vi "Init_Robot_State.vi"(8 "error in (no error)":errorcluster) -> (0 "error out":errorcluster, 3 "MotionCtlLoop_Data":T1)   [LabVIEW 2017]
doc: "Initialise robot's position and forward & rotation velocity to 0"
uses:
  Ctl/MotionControlLoop_Data_Cluster.ctl
  Ctl/Current_Position.ctl
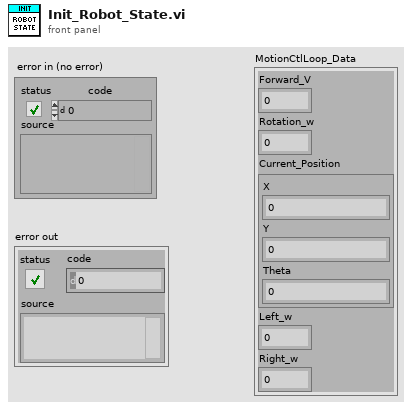
[diagram p1: front panel]
types:
  T1 = typedef "MotionControlLoop_Data_Cluster.ctl" = cluster{"Forward_V":dbl, "Rotation_w":dbl, "Current_Position":T2, "Left_w":dbl, "Right_w":dbl}
  T2 = typedef "Current_Position.ctl" = cluster{"X":dbl, "Y":dbl, "Theta":dbl}
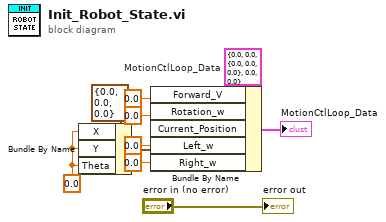
[diagram p0: block diagram]
diagram:
  w10 = 0.0 ("X")
  w2 = T1 {"Forward_V"=0.0, "Rotation_w"=0.0, "Current_Position"={"X"=0.0, "Y"=0.0, "Theta"=0.0}, "Left_w"=0.0, "Right_w"=0.0}  # MotionCtlLoop_Data
  n1 = Bundle By Name(cluster=T2 {"X"=0.0, "Y"=0.0, "Theta"=0.0} ("Current_Position"), "X"=w10, "Y"=w10, "Theta"=w10) -> (w9:T2)
  n2 = Bundle By Name(cluster=w2, "Forward_V"=0.0, "Rotation_w"=0.0, "Current_Position"=w9, "Left_w"=0.0, "Right_w"=0.0) -> (→"MotionCtlLoop_Data":T1)
  "error out" <- "error in (no error)"
